vi "online_wavlength_lock_Pro800.vi"(4 "Device":refnum<visa-resource-name>="Pro8000", 6 "Settings In":T1={"Module"=enum."On Line TEC", "OnLineTEC"=23.261520000000402, "OnLineLD"=0.1722} {"OnLineLD" min=0.0 max=0.175 step=0.001 format="%.3p"; "OnLineTEC" min=0.0 max=30.0 step=0.1 format="%.3g"}, 7 "Lambda On Set (nm)":dbl=828.198 format="%.5f", 8 "step_size":dbl=0.00025 format="%#_6p") -> (1 "Wavelength Lock Online":bool=TRUE, 2 "Lambda On Read (nm)":dbl=828.1980271680263 format="%.5f")   [LabVIEW 2012]
uses:
  <vilib>/DAQmx/write.llb/DAQmx Write (Digital 1D Bool NChan 1Samp 1Line).vi
  <vilib>/DAQmx/miscellaneous.llb/DAQmx Fill In Error Info.vi
  Shared Telescope WV DIAL Code/bristol/CLDevIFace.dll
panel:
  in  "Online_Tol":dbl=5e-05 format="%#_15g"
  out "WL_Difference":dbl=2.7168026349499996e-05 format="%#_3e"
  in  "Cancel online":bool
  in  "Bristol In":i32=5
  out "Bristol Out":i32
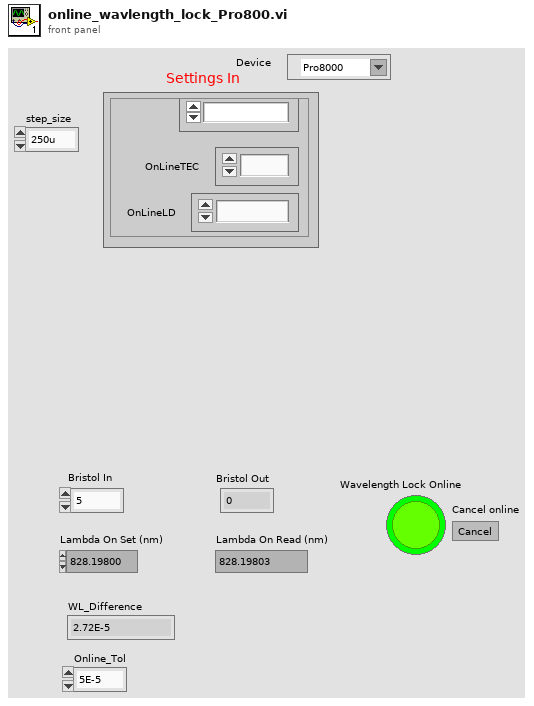
[diagram p1: front panel]
types:
  T1 = cluster{"Module":enum16{"On Line TEC", "On Line LD"}, "OnLineTEC":dbl, "OnLineLD":dbl}
  T2 = enum16{"Open_TL", "Close_TL", "Verify_ID", "TEC_Sensor", "SET", "READ", "ON", "OFF", "Read_Status"}
  T3 = enum16{"On Line TEC", "On Line LD", "Off Line TEC", "Off Line LD", "Etalon TEC", "TSOA TEC"}
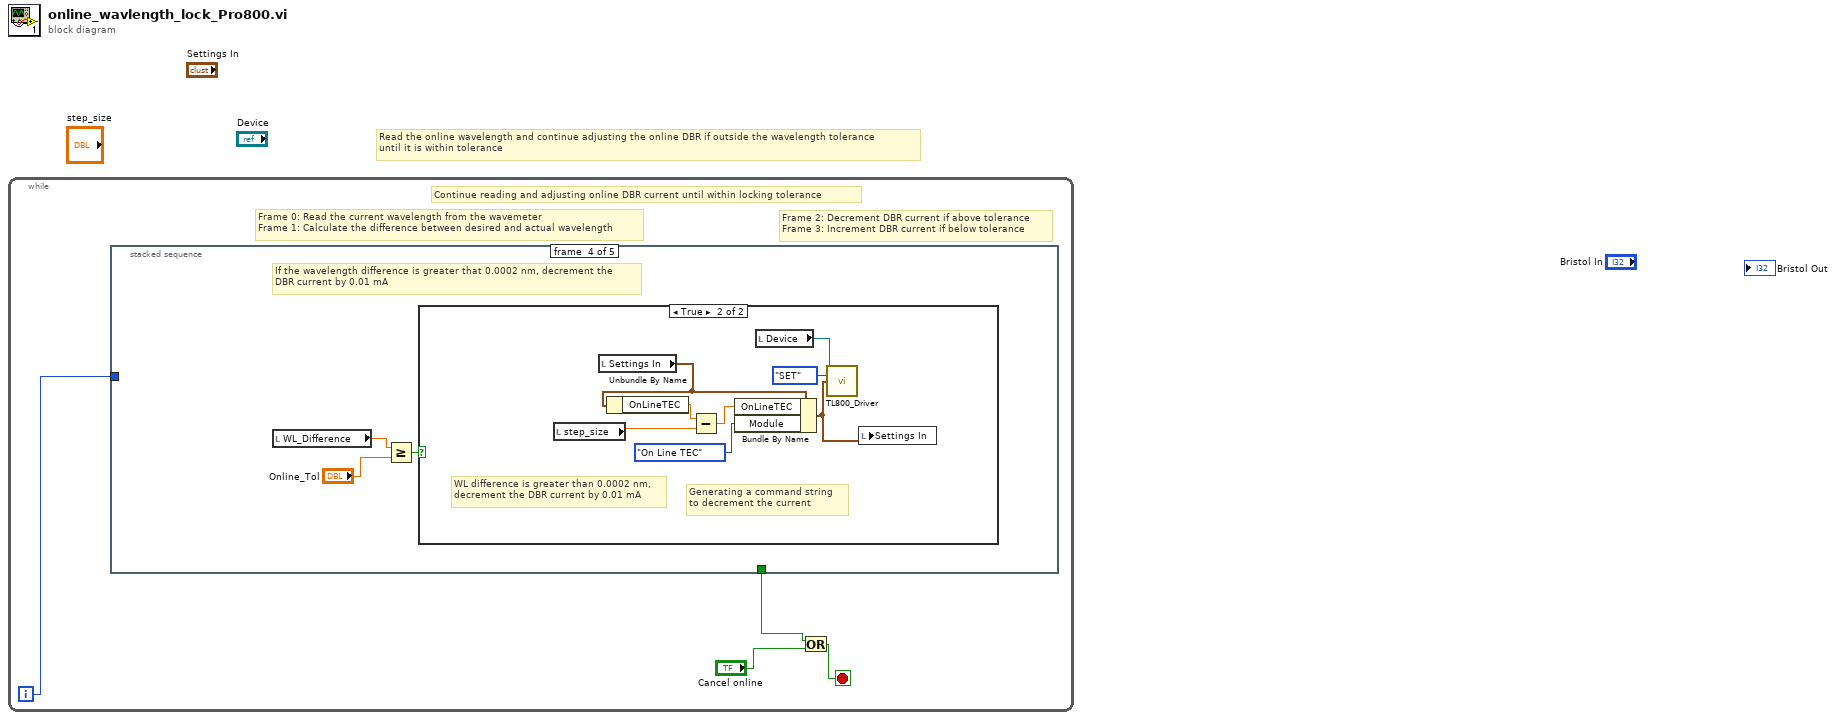
[diagram p0: block diagram]
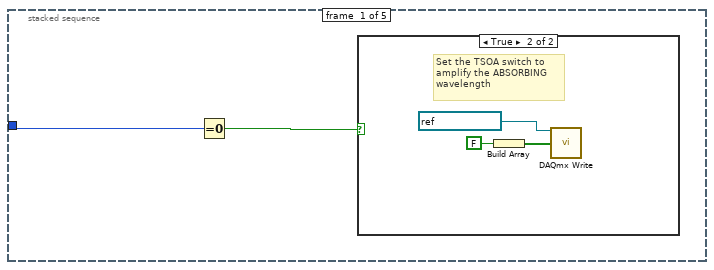
[diagram p2: hidden frame]
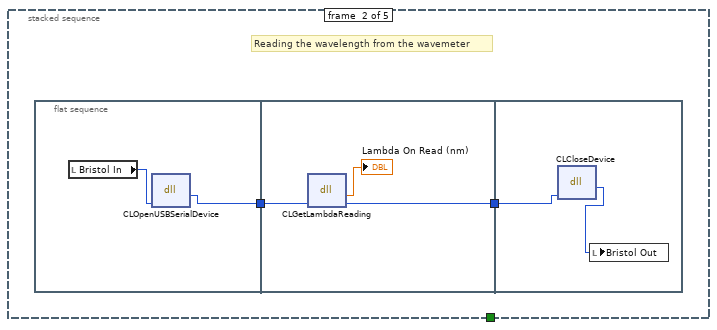
[diagram p4: hidden frame]
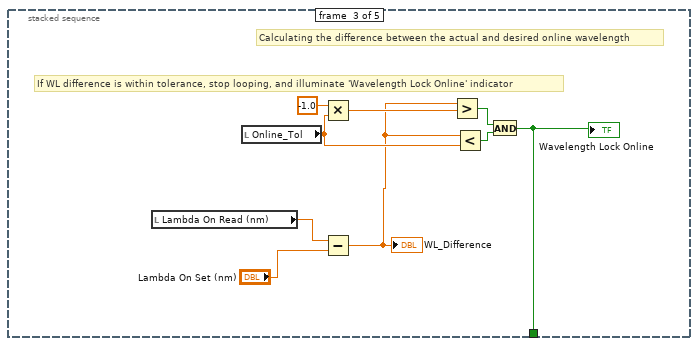
[diagram p5: hidden frame]
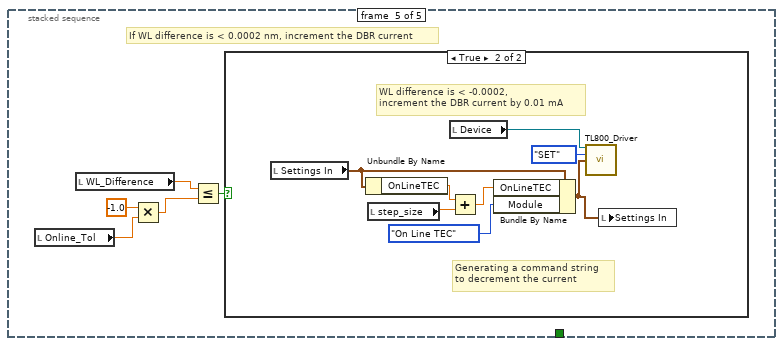
[diagram p7: hidden frame]
diagram:
  # "Read the online wavelength and continue adjusting the online DBR if outside the wavelength tolerance\nuntil it is within tolerance"
  n1 = while {
    i -> [w4]
    stop <- w1 stop-if-true
    # "Frame 2: Decrement DBR current if above tolerance\nFrame 3: Increment DBR current if below tolerance"
    # "Frame 0: Read the current wavelength from the wavemeter\nFrame 1: Calculate the difference between desired and actual wavelength"
    # "Continue reading and adjusting online DBR current until within locking tolerance"
    n2 = stacked-sequence {
      tunnel: w4 -> [w6 _ _ _ _]
      tunnel: [_ _ w19 _ _] -> w2
      frame #0 {
        n3 = Equal To 0?(x=w6) -> (x = 0?=w5:bool)
        n4 = case shown="True" w5 {
          frame False {
          }
          frame True {
            # "Set the TSOA switch to\namplify the ABSORBING\nwavelength"
            n5 = Build Array(FALSE ("Boolean")) -> (w7:bool[])
            n6 = call-poly <vilib>:"DAQmx Write.vi"("task/channels in"=refnum<k21> "BristolWM", "data"=w7) -> ()  [unwired: 11 in, 3 out]
          }
        }
      }
      frame #1 {
        # "Reading the wavelength from the wavemeter"
        n7 = flat-sequence {
          tunnel: [w12] -> w11
          tunnel: w11 -> [w15]
          tunnel: [w14] -> w10
          tunnel: w10 -> [w18]
          frame #0 {
            n8 = local read "Bristol In"() -> (w13:i32)
            n9 = dll-call lib="C:/Users/H2ODial/Desktop/Shared Telescope WV DIAL Code/bristol/CLDevIface.dll" fn="CLOpenUSBSerialDevice"("commPort"=w13) -> ("return type"=w12:i32)  [unwired: 4 in, 2 out]
          }
          frame #1 {
            n10 = dll-call lib="C:/Users/H2ODial/Desktop/Shared Telescope WV DIAL Code/bristol/CLDevIface.dll" fn="CLGetLambdaReading"("devHandle"=w15) -> ("return type"=→"Lambda On Read (nm)":dbl, "devHandle"=w14:i32)  [unwired: 3 in, 2 out]
          }
          frame #2 {
            n11 = dll-call lib="C:/Users/H2ODial/Desktop/Shared Telescope WV DIAL Code/bristol/CLDevIface.dll" fn="CLCloseDevice"("commPort"=w18) -> ("return type"=w17:i32)  [unwired: 4 in, 2 out]
            n12 = local write "Bristol Out"(w17) -> ()
          }
        }
      }
      frame #2 {
        # "If WL difference is within tolerance, stop looping, and illuminate 'Wavelength Lock Online' indicator"
        # "Calculating the difference between the actual and desired online wavelength"
        n13 = local read "Lambda On Read (nm)"() -> (w27:dbl)
        n14 = local read "Online_Tol"() -> (w24:dbl)
        n15 = Multiply(x=-1.0, y=w24) -> (x*y=w25:dbl)
        n16 = Subtract(x=w27, y="Lambda On Set (nm)") -> (x-y=w20:dbl)
        "WL_Difference" <- w20
        n17 = Greater?(x=w20, y=w25) -> (0:w21:bool)
        n18 = Less?(x=w20, y=w24) -> (x < y?=w22:bool)
        n19 = And(x=w21, y=w22) -> (x .and. y?=w19:bool)
        "Wavelength Lock Online" <- w19
      }
      frame #3 {
        # "If the wavelength difference is greater that 0.0002 nm, decrement the \nDBR current by 0.01 mA"
        n20 = local read "WL_Difference"() -> (w30:dbl)
        n21 = Greater Or Equal?(x=w30, y="Online_Tol") -> (x >= y?=w29:bool)
        n22 = case shown="True" w29 {
          frame False {
            # "Wavelength difference is not greater than 0.0002 nm, do nothing"
          }
          frame True {
            # "Generating a command string\nto decrement the current"
            # "WL difference is greater than 0.0002 nm,\ndecrement the DBR current by 0.01 mA"
            n23 = local read "step_size"() -> (w35:dbl)
            n24 = local read "Settings In"() -> (w34:T1)
            n25 = Unbundle By Name(w34) -> ("OnLineTEC"=w37:dbl)
            n26 = Subtract(x=w37, y=w35) -> (x-y=w36:dbl)
            n27 = Bundle By Name(cluster=w34, "OnLineTEC"=w36, "Module"=T3."On Line TEC") -> (w32:T1)
            n28 = local read "Device"() -> (w33:refnum<visa-resource-name>)
            n29 = call "TL800_Driver.vi"("Device In"=w33, "Commands"=T2."SET", "Settings"=w32) -> ()  [unwired: 9 in, 4 out]
            n30 = local write "Settings In"(w32) -> ()
          }
        }
      }
      frame #4 {
        # "If WL difference is < 0.0002 nm, increment the DBR current"
        n31 = local read "Online_Tol"() -> (w40:dbl)
        n32 = local read "WL_Difference"() -> (w43:dbl)
        n33 = Multiply(x=-1.0, y=w40) -> (x*y=w39:dbl)
        n34 = Less Or Equal?(x=w43, y=w39) -> (x <= y?=w42:bool)
        n35 = case shown="True" w42 {
          frame False {
            # "WL difference is no <= to -0.0002 nm, do nothing"
          }
          frame True {
            # "WL difference is < -0.0002,\nincrement the DBR current by 0.01 mA"
            # "Generating a command string\nto decrement the current"
            n36 = local read "Settings In"() -> (w51:T1)
            n37 = Unbundle By Name(w51) -> ("OnLineTEC"=w49:dbl)
            n38 = local read "step_size"() -> (w45:dbl)
            n39 = local read "Device"() -> (w46:refnum<visa-resource-name>)
            n40 = Add(x=w49, y=w45) -> (x+y=w48:dbl)
            n41 = Bundle By Name(cluster=w51, "OnLineTEC"=w48, "Module"=T3."On Line TEC") -> (w44:T1)
            n42 = call "TL800_Driver.vi"("Device In"=w46, "Commands"=T2."SET", "Settings"=w44) -> ()  [unwired: 9 in, 4 out]
            n43 = local write "Settings In"(w44) -> ()
          }
        }
      }
    }
    n44 = Or(x=w2, y="Cancel online") -> (x .or. y?=w1:bool)
  }
